vi "Vision Research Phantom Series PhFile PhSetCineInfo.vi"(0 "CH [in]":u32=1, 1 "InfName [in]":T1 items=["GCI_CFA"=0, "GCI_FRAMERATE"=1, "GCI_EXPOSURE"=2, "GCI_AUTOEXPOSURE"=3, "GCI_REALBPP"=4, "GCI_CAMERASERIAL"=5, "GCI_HEADSERIAL0"=6, "GCI_HEADSERIAL1"=7, "GCI_HEADSERIAL2"=8, "GCI_HEADSERIAL3"=9, "GCI_TRIGTIMESEC"=10, "GCI_TRIGTIMEFR"=11, "GCI_ISFILECINE"=12, "GCI_IS16BPPCINE"=13, "GCI_ISCOLORCINE"=14, "GCI_ISMULTIHEADCINE"=15, "GCI_EXPOSURENS"=16, "GCI_EDREXPOSURENS"=17, "GCI_FRAMEDELAYNS"=19, "GCI_FROMFILETYPE"=20, "GCI_COMPRESSION"=21, "GCI_CAMERAVERSION"=22, "GCI_ROTATE"=23, "GCI_IMWIDTH"=24, "GCI_IMHEIGHT"=25, "GCI_IMWIDTHACQ"=26, "GCI_IMHEIGHTACQ"=27, "GCI_POSTTRIGGER"=28, "GCI_IMAGECOUNT"=29, "GCI_TOTALIMAGECOUNT"=30, "GCI_TRIGFRAME"=31, "GCI_AUTOEXPLEVEL"=32, "GCI_AUTOEXPTOP"=33, "GCI_AUTOEXPLEFT"=34, "GCI_AUTOEXPBOTTOM"=35, "GCI_AUTOEXPRIGHT"=36, "GCI_RECORDINGTIMEZONE"=37, "GCI_FIRSTIMAGENO"=38, "GCI_FIRSTMOVIEIMAGE"=39, "GCI_CINENAME"=40, "GCI_FRPSTEPS"=100, "GCI_FRP1X"=101, "GCI_FRP1Y"=102, "GCI_FRP2X"=103, "GCI_FRP2Y"=104, "GCI_FRP3X"=105, "GCI_FRP3Y"=106, "GCI_FRP4X"=107, "GCI_FRP4Y"=108, "GCI_WRITEERR"=109, "GCI_LENSDESCRIPTION"=110, "GCI_LENSAPERATURE"=111, "GCI_LENSFOCALLENGTH"=112, "GCI_WB"=200, "GCI_WBVIEW"=201, "GCI_BRIGHT"=202, "GCI_CONTRAST"=203, "GCI_GAMMA"=204, "GCI_GAMMAR"=223, "GCI_GAMMAB"=224, "GCI_SATURATION"=205, "GCI_HUE"=206, "GCI_FLIPH"=207, "GCI_FLIPV"=208, "GCI_FILTERCODE"=209, "GCI_IMFILTER"=210, "GCI_INTALGO"=211, "GCI_PEDESTALR"=212, "GCI_PEDESTALG"=213, "GCI_PEDESTALB"=214, "GCI_FLARE"=225, "GCI_CHROMA"=226, "GCI_TONE"=227, "GCI_ENABLEMATRICES"=228, "GCI_USERMATRIX"=229, "GCI_RESAMPLEACTIVE"=215, "GCI_RESAMPLEWIDTH"=216, "GCI_RESAMPLEHEIGHT"=217, "GCI_CROPACTIVE"=218, "GCI_CROPRECTANGLE"=219, "GCI_OFFSET16_8"=220, "GCI_GAIN16_8"=221, "GCI_DEMOSAICINGFUNCPTR"=222, "GCI_VFLIPVIEWACTIVE"=300, "GCI_MAXIMGSIZE"=400, "GCI_FRPIMGNOARRAY"=450, "GCI_FRPRATEARRAY"=451, "GCI_FRPSHAPEARRAY"=452, "GCI_TRIGTC"=470, "GCI_TRIGTCU"=471, "GCI_PBRATE"=472, "GCI_TCRATE"=473, "GCI_SAVERANGE"=500, "GCI_SAVEFILENAME"=501, "GCI_SAVEFILETYPE"=502, "GCI_SAVE16BIT"=503, "GCI_SAVEPACKED"=504, "GCI_SAVEXML"=505, "GCI_SAVESTAMPTIME"=506, "GCI_SAVEAVIFRAMERATE"=520, "GCI_SAVEAVICOMPRESSORLIST"=521, "GCI_SAVEAVICOMPRESSORINDEX"=522, "GCI_SAVEDPXLSB"=530, "GCI_SAVEDPXTO10BPS"=531, "GCI_SAVEDPXDATAPACKING"=532, "GCI_SAVEDPX10BITLOG"=533, "GCI_SAVEDPXEXPORTLOGLUT"=534, "GCI_SAVEDPX10BITLOGREFWHITE"=535, "GCI_SAVEDPX10BITLOGREFBLACK"=536, "GCI_SAVEDPX10BITLOGGAMMA"=537, "GCI_SAVEDPX10BITLOGFILMGAMMA"=538, "GCI_SAVEQTPLAYBACKRATE"=550, "GCI_SAVECCIQUALITY"=560, "GCI_UNCALIBRATEDIMAGE"=600, "GCI_NOPROCESSING"=601, "GCI_BADPIXELREPAIR"=602], 2 "pInfVal [in]":i32, 5 "Error In (no error)":errorcluster) -> (14 "CH [out]":u32, 15 "pInfVal [out]":i32, 19 "Error Out":errorcluster)   [LabVIEW 2013, in "VRI.lvlib"]
doc: "PhSetCineInfo\nHRESULT PhSetCineInfo(CINEHANDLE CH, UINT InfName, PVOID pInfVal);\n\nParameters\nCH [in]\n The cine the information is set for.\nInfName [in]\n Numerical value identifying the parameter to be set.\npInfVal [in, out]\n Input: pointer containing the value to be set.\n Output: pointer containing accepted value.\n\nReturn Value\nThe function returns ERR_Ok in case of success or an error code, otherwise. To get extended error information call PhGetErrorMessage.\n\nRemarks\nIt is the main function used for setting cine parameters such as image processing parameters or saving options. It requires as input data a cine handle, a numerical value indicating what parameter is to be modified and the actual value to be set.\nPlease note that the last parameter must be passed by reference! The function will return back to the caller the value actually accepted for the specified cine parameter.\nCheck Appendix 1 for a complete list of selectors PhSetCineInfo accepts.\n\nRequired Header\nPhFile.h"
uses:
  VRI.lvlib
  _Type Defs/PhFile InfName.ctl
  Phantom DLLs/PhFile.Dll
panel:
  # "For instructions on the use of this VI, press Ctrl+H to display the help window and move the mouse over the icon, controls, and indicators"
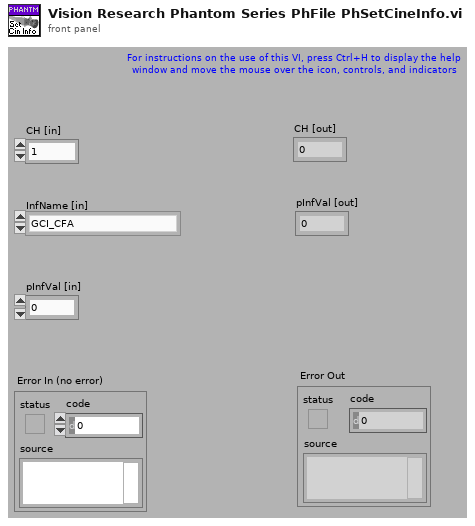
[diagram p1: front panel]
types:
  T1 = typedef "VRI.lvlib/PhFile InfName.ctl" = u32
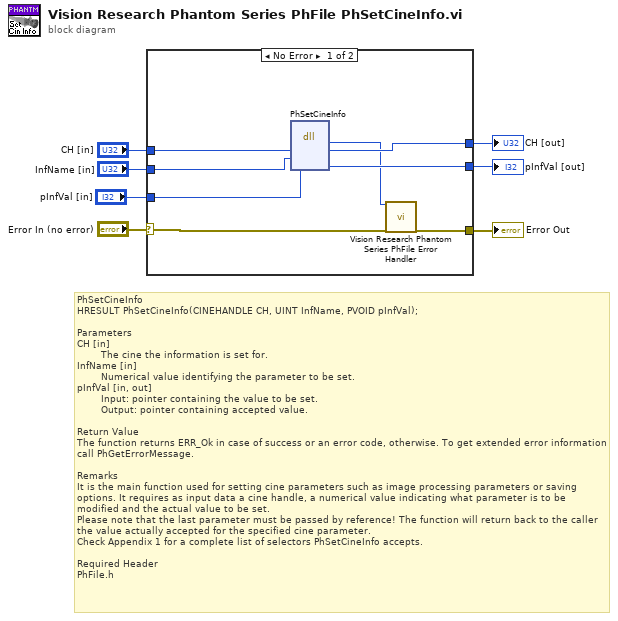
[diagram p0: block diagram]
diagram:
  # "PhSetCineInfo\nHRESULT PhSetCineInfo(CINEHANDLE CH, UINT InfName, PVOID pInfVal);\n\nParameters\nCH [in]\n\t       The cine the information is set for.\nInfName [in]\n\t       Numerical value identifying the parameter to be set.\npInfVal [in, out]\n\t       Input: pointer containing the value to be set.\n\t       Output: pointer containing accepted value.\n\nReturn Value\nThe function returns ERR_Ok in case of success or an error code, otherwise. To get extended error information call PhGetErrorMessage.\n\nRemarks\nIt is the main function used for setting cine parameters such as image processing parameters or saving options. It requires as input data a cine handle, a numerical value indicating what parameter is to be modified and the actual value to be set.\nPlease note that the last parameter must be passed by reference! The function will return back to the caller the value actually accepted for the specified cine parameter.\nCheck Appendix 1 for a complete list of selectors PhSetCineInfo accepts.\n\nRequired Header\nPhFile.h"
  n1 = case shown="No Error" "Error In (no error)" {
    selector: "Error In (no error)" -> [w15 w18]
    tunnel: [w14 w18] -> w6
    tunnel: "CH [in]" -> [w13 w16]
    tunnel: "InfName [in]" -> [w12 _]
    tunnel: "pInfVal [in]" -> [w11 w17]
    tunnel: [w10 w17] -> w2
    tunnel: [w9 w16] -> w1
    frame No Error {
      n2 = dll-call lib="C:/Projects/SDK/64-bit/Vision Research Phantom Series Labview Driver/Phantom DLLs/PhFile.dll" fn="PhSetCineInfo"("CH"=w13, "InfName"=w12, "pInfVal"=w11) -> ("HRESULT"=w8:i32, "CH"=w9:u32, "pInfVal"=w10:i32)  [unwired: 4 in, 2 out]
      n3 = call "Vision Research Phantom Series PhFile Error Handler.vi"("Error Code (0)"=w8, "Error In (no error)"=w15) -> ("Error Out"=w14:errorcluster)  [unwired: 17 out]
    }
    frame Error {
    }
  }
  "Error Out" <- w6
  "pInfVal [out]" <- w2
  "CH [out]" <- w1
